vi "fpga_idx2target.vi"(5 "delta":T1, 7 "initial position":T1, 11 "idx":i16) -> (3 "target":T1)   [LabVIEW 2021]
doc: "Calculate target position from index."
uses:
  fpga_dtype_sgl_8ch.ctl
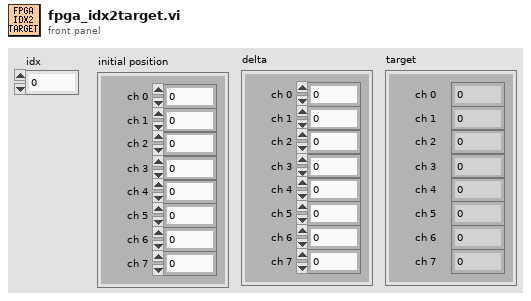
[diagram p1: front panel]
types:
  T1 = typedef "fpga_dtype_sgl_8ch.ctl" = cluster{"ch 0":sgl, "ch 1":sgl, "ch 2":sgl, "ch 3":sgl, "ch 4":sgl, "ch 5":sgl, "ch 6":sgl, "ch 7":sgl}
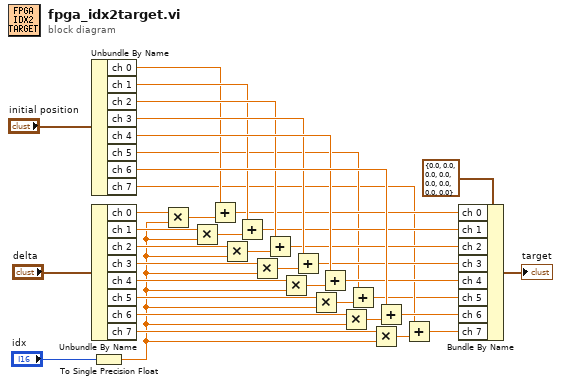
[diagram p0: block diagram]
diagram:
  n1 = Unbundle By Name("initial position") -> ("ch 0"=w14:sgl, "ch 1"=w15:sgl, "ch 2"=w16:sgl, "ch 3"=w17:sgl, "ch 4"=w18:sgl, "ch 5"=w8:sgl, "ch 6"=w19:sgl, "ch 7"=w6:sgl)
  n2 = Unbundle By Name("delta") -> ("ch 0"=w37:sgl, "ch 1"=w35:sgl, "ch 2"=w34:sgl, "ch 3"=w33:sgl, "ch 4"=w32:sgl, "ch 5"=w31:sgl, "ch 6"=w30:sgl, "ch 7"=w36:sgl)
  n3 = To Single Precision Float(number="idx") -> (single precision float=w28:sgl)
  n4 = Multiply(x=w37, y=w28) -> (x*y=w27:sgl)
  n5 = Multiply(x=w35, y=w28) -> (x*y=w25:sgl)
  n6 = Add(x=w14, y=w27) -> (x+y=w13:sgl)
  n7 = Multiply(x=w34, y=w28) -> (x*y=w24:sgl)
  n8 = Add(x=w15, y=w25) -> (x+y=w12:sgl)
  n9 = Multiply(x=w33, y=w28) -> (x*y=w23:sgl)
  n10 = Add(x=w16, y=w24) -> (x+y=w11:sgl)
  n11 = Multiply(x=w32, y=w28) -> (x*y=w22:sgl)
  n12 = Add(x=w17, y=w23) -> (x+y=w10:sgl)
  n13 = Multiply(x=w31, y=w28) -> (x*y=w21:sgl)
  n14 = Add(x=w18, y=w22) -> (x+y=w9:sgl)
  n15 = Multiply(x=w30, y=w28) -> (x*y=w20:sgl)
  n16 = Add(x=w8, y=w21) -> (x+y=w2:sgl)
  n17 = Multiply(x=w36, y=w28) -> (x*y=w26:sgl)
  n18 = Add(x=w19, y=w20) -> (x+y=w7:sgl)
  n19 = Add(x=w6, y=w26) -> (x+y=w1:sgl)
  n20 = Bundle By Name(cluster=T1 {"ch 0"=0.0, "ch 1"=0.0, "ch 2"=0.0, "ch 3"=0.0, "ch 4"=0.0, "ch 5"=0.0, "ch 6"=0.0, "ch 7"=0.0} ("sgl 8ch"), "ch 0"=w13, "ch 1"=w12, "ch 2"=w11, "ch 3"=w10, "ch 4"=w9, "ch 5"=w2, "ch 6"=w7, "ch 7"=w1) -> (→"target":T1)
